vi "Spantabellenanzeige.vi"(8 "error in (no error)":errorcluster caption="Fehler (Eingang, kein Fehler)") -> (0 "error out":errorcluster caption="Fehler (Ausgang)", 3 "SpanTabelle":T1[][](array[typedef]))   [LabVIEW 2020, in "Linearisierung v2.lvlib"]
uses:
  Linearisierung v2.lvlib
  Visualisierungs Elemente/String - Ausgabefeld.ctl
  Seiten/FT-IR/Span/Aktion FGV Span.ctl
  Messdaten/Aktionen FGV Messdaten.ctl
  Seiten/FT-IR/FGV FT-IR Gasliste Aktionen.ctl
  Seiten/FT-IR/Aktionen EVID-Codes.ctl
  Seiten/FT-IR/Span/Spanfaktor.lvlib
  Messdaten/Messdaten.lvlib
  Seiten/FT-IR/FT-IR.lvlib
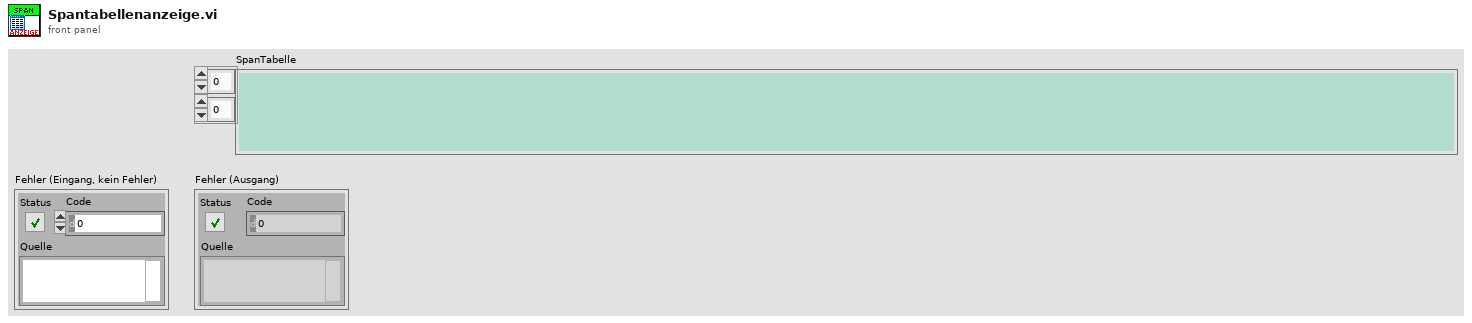
[diagram p1: front panel]
types:
  T1 = typedef "String - Ausgabefeld.ctl" = string
  T2 = typedef "FT-IR.lvlib/Aktionen EVID-Codes.ctl" = enum16{"lesen", "setzen", "laden", "speichern", "1Hz/5Hz", "Smoothing", "Rolling Average"}
  T3 = typedef "FT-IR.lvlib/FGV FT-IR Gasliste Aktionen.ctl" = enum16{"lesen", "Gasliste FT-IR", "Gasliste ausgelesen", "laden", "speichern", "löschen"}
  T4 = typedef "Messdaten.lvlib/Aktionen FGV Messdaten.ctl" = enum16{"lesen", "schreiben", "löschen", "Mittelwerte", "Komponente"}
  T5 = typedef "FT-IR.lvlib/Spanfaktor.lvlib/Aktion FGV Span.ctl" = enum16{"lesen", "Span", "Seite aktiv", "Offset", "FGV aktualisiert", "Aktualisierung aufheben"}
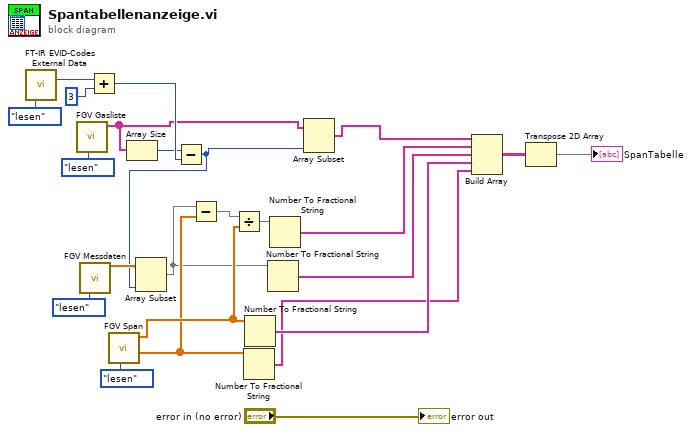
[diagram p0: block diagram]
diagram:
  n1 = call "FT-IR EVID-Codes External Data.vi"("Aktionen"=Aktionen_EVID-Codes."lesen") -> ("Anzahl"=w17:i32)  [unwired: 9 in, 5 out]
  n2 = call "FGV Gasliste.vi"("Aktionen"=FGV_FT-IR_Gasliste_Aktionen."lesen") -> ("Aktuelle Gasliste FT-IR"=w6:T1[])  [unwired: 8 in, 2 out]
  n3 = call "FGV Messdaten.vi"("Aktionen"=Aktionen_FGV_Messdaten."lesen") -> ("Aktuelle Messwerte"=w4:sgl[])  [unwired: 6 in, 8 out]
  n4 = Add(x=w17, y=3) -> (x+y=w15:i32)
  n5 = call "FGV Span.vi"("Aktion"=Aktion_FGV_Span."lesen") -> ("Offset"=w21:sgl[], "Span"=w22:sgl[])  [unwired: 7 in, 2 out]
  n6 = Array Size(array=w6) -> (size(s)=w14:i32)
  n7 = Subtract(x=w14, y=w15) -> (x-y=w2:i32)
  n8 = Array Subset(array=w4, length=w2) -> (w3:sgl[])  [unwired: 1 in]
  n9 = Subtract(x=w3, y=w21) -> (x-y=w20:sgl[])
  n10 = Divide(x=w20, y=w22) -> (x/y=w19:sgl[])
  n11 = Number To Fractional String(number=w21) -> (F-format string=w9:string[])  [unwired: 3 in]
  n12 = Number To Fractional String(number=w22) -> (F-format string=w10:string[])  [unwired: 3 in]
  n13 = Number To Fractional String(number=w3) -> (F-format string=w11:string[])  [unwired: 3 in]
  n14 = Number To Fractional String(number=w19) -> (F-format string=w12:string[])  [unwired: 3 in]
  n15 = Array Subset(array=w6, length=w2) -> (w5:T1[])  [unwired: 1 in]
  n16 = Build Array(w5, w12, w11, w10, w9) -> (w8:T1[][])
  n17 = Transpose 2D Array(2D array=w8) -> (transposed array=→"SpanTabelle":T1[][])
  "error out" <- "error in (no error)"
